vi "FPGA_controlled VI.vi"() -> ()   [LabVIEW 2020]
uses:
  <vilib>/eio/EIONode/EIONode.xnode
  <vilib>/rvi/eio/common/nirviEmuTemplateMethod_errors.vi
panel:
  in  "stop":bool
  in  "Mod4/AO0":fxp<+/-,20,5>
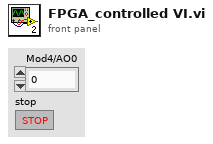
[diagram p1: front panel]
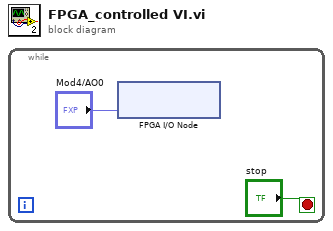
[diagram p0: block diagram]
diagram:
  n1 = while {
    stop <- "stop" stop-if-true
    n2 = xnode "FPGA I/O Node"("Mod4/AO0"="Mod4/AO0") -> ()  [unwired: 1 in, 1 out]
  }
